vi "Pour.vi"(8 "error in (no error)":errorcluster, 11 "Ale in":refnum<class "Ale.lvclass">) -> (0 "error out":errorcluster, 3 "Ale out":refnum<class "Ale.lvclass">)   [LabVIEW 2011, in "Ale.lvclass"]
uses:
  Ale.lvclass
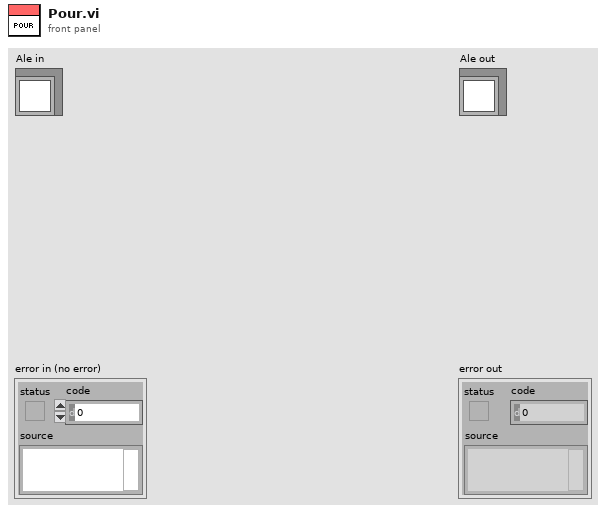
[diagram p1: front panel]
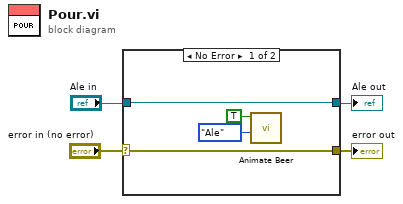
[diagram p0: block diagram]
diagram:
  n1 = case shown="No Error" "error in (no error)" {
    selector: "error in (no error)" -> [w7 w9]
    tunnel: "Ale in" -> [w8 w10]
    tunnel: [w8 w10] -> w3
    tunnel: [w7 w9] -> w2
    frame No Error {
      n2 = call "Animate Beer.vi"("Type"=enum16{"Lager", "Ale", "Guiness"}."Ale", "Tilt"=TRUE) -> ()  [unwired: 10 in]
    }
    frame Error {
    }
  }
  "error out" <- w2
  "Ale out" <- w3
